vi "Launcher.vi"() -> ()   [LabVIEW 2022 SP3]
doc: "JKI State Machine Objects (SMO) 1.0.0.5\nJKI - JKI\nCopyright (c) 2016, JKI"
uses:
  002_SRC/Splashy/Splashy.lvclass
  C:/Program Files (x86)/National Instruments/LabVIEW 2022/vi.lib/JKI/JKI SMO/SMO/SMO.lvclass
  C:/Program Files (x86)/National Instruments/LabVIEW 2022/vi.lib/JKI/JKI SMO/SMO.UI/SMO.UI.lvclass
  002_SRC/GUI/GUI.lvclass
  <vilib>/JKI/JKI SMO/SMO/SMO.lvclass/SMO.ctl
  <vilib>/JKI/JKI SMO/SMO.UI/SMO.UI.lvclass/SMO.UI.ctl
  <vilib>/JKI/JKI SMO/SMO/Typedefs/SMOState --Enum.ctl
  f04c7903-df52-4a90-82d6-ebb4e2f21dec.vi
  <vilib>/JKI/JKI SMO/SMO/Private/ReftoDVR--SMO.vi
  <vilib>/JKI/JKI SMO/SMO.UI/SMO.UI.ReftoDVR.vi
  <vilib>/JKI/JKI SMO/SMO/SMO.lvclass
  <vilib>/JKI/JKI SMO/SMO.UI/SMO.UI.lvclass
  C:/Users/uib01493/Desktop/001_Final_Project/002_SRC/Splashy/Splashy.lvclass
  C:/Users/uib01493/Desktop/001_Final_Project/002_SRC/GUI/GUI.lvclass
panel:
  out "error out":errorcluster
  in  "Stop":bool
  # "SMO Splash Test Launcher"
  # "For instructions on how to use the JKI State Machine Objects, examples and video tutorials, visit:\nhttp://jki.net/state-machine-objects/\n\nJKI State Machine Objects™\nhttp://jki.net/state-machine-objects/\nCopyright (C) 2005-2015, JKI <info@jki.net>\nALL RIGHTS RESERVED"
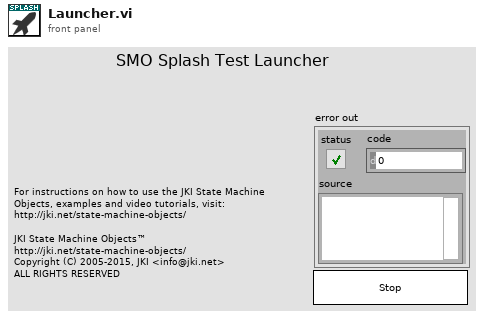
[diagram p1: front panel]
types:
  T1 = enum32{"Invalid", "Standard", "Closed", "Hidden", "Minimized", "Maximized"}
  T2 = typedef "SMO.lvclass/Public Events.ctl" = cluster{"Error":refnum<user-event>, "State":refnum<user-event>, "Reserve State":refnum<user-event>}
  T3 = typedef "SMO.UI.lvclass/PublicEvents--Cluster.ctl" = cluster{"UI Hidden":refnum<user-event>, "UI State":refnum<user-event>}
  T4 = typedef "SMO.lvclass/SMOState --Enum.ctl" = enum16{"unknown", "Created", "Started", "Stopped"}
  T5 = typedef "GUI.lvclass/PublicEvents--Cluster.ctl" = cluster{"Data Changed":refnum<user-event>}
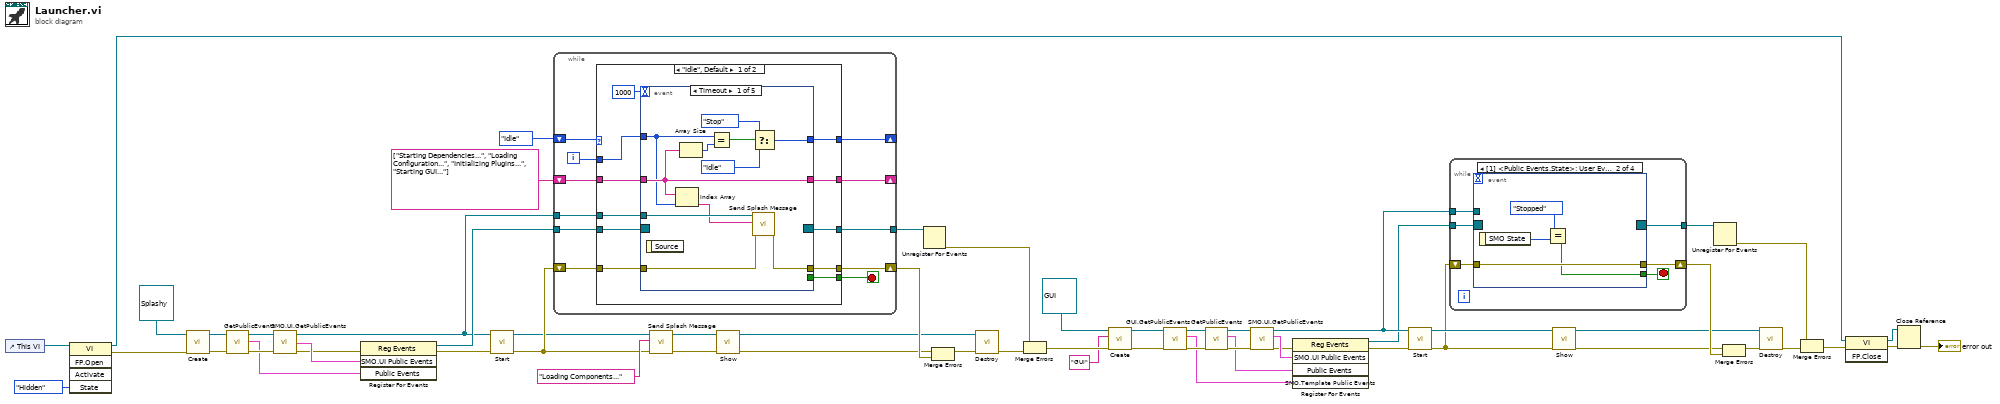
[diagram p0: block diagram]
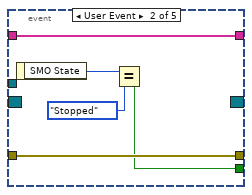
[diagram p2: hidden frame]
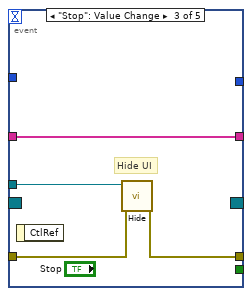
[diagram p3: hidden frame]
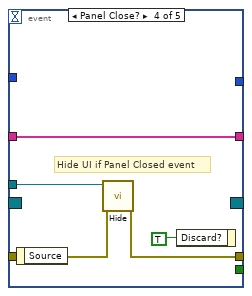
[diagram p4: hidden frame]
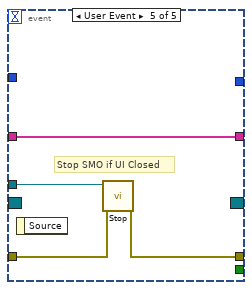
[diagram p5: hidden frame]
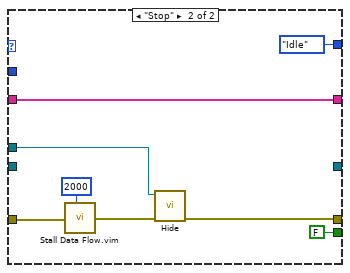
[diagram p6: hidden frame]
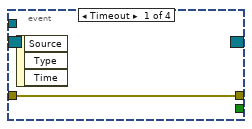
[diagram p7: hidden frame]
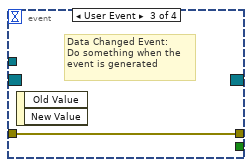
[diagram p8: hidden frame]
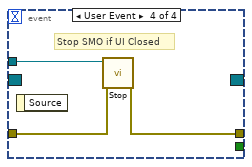
[diagram p9: hidden frame]
diagram:
  n1 = control-ref of="This VI"() -> (w8:refnum<vi>)
  n2 = invoke class="VI" method="FP.Open"(reference=w8, "State"=T1."Hidden") -> (reference out=w4:refnum<vi>, error out=w35:errorcluster)  [unwired: 3 in, 3 out]
  n3 = call <vilib>:"Create.vi"("error in (no error)"=w35, "SMO"=refnum<class "Splashy.lvclass"> refnum ("SMO.Template.lvclass")) -> ("error out"=w41:errorcluster, "SMO out"=w43:refnum<class "Splashy.lvclass">)  [unwired: 7 in, 1 out]
  n4 = call <vilib>:"GetPublicEvents.vi"("error in (no error)"=w41, "SMO"=w43) -> ("error out"=w40:errorcluster, "Public Events"=w39:T2, "SMO out"=w42:refnum<class "Splashy.lvclass">)  [unwired: 7 in]
  n5 = call <vilib>:"SMO.UI.GetPublicEvents.vi"("error in (no error)"=w40, "SMO.UI"=w42) -> ("error out"=w45:errorcluster, "SMO.UI Public Events"=w46:T3, "SMO.UI out"=w37:refnum<class "Splashy.lvclass">)  [unwired: 7 in]
  n6 = register-events(error in=w45, w46, w39) -> (reference out=w38:refnum<event-registration>, error out=w44:errorcluster)  [unwired: 1 in]
  n7 = call <vilib>:"Start.vi"("error in (no error)"=w44, "SMO"=w37) -> ("error out"=w50:errorcluster, "SMO out"=w47:refnum<class "Splashy.lvclass">)  [unwired: 8 in]
  n8 = while {
    shift-right: [w68] -> w57
    shift-left: w50 -> [w67]
    tunnel: w38 -> [w66]
    tunnel: [w65] -> w58
    tunnel: w37 -> [w64]
    shift-right: [w61] -> _
    shift-left: string[] ["Starting Dependencies...", "Loading Configuration...", "Initializing Plugins...", "Starting GUI..."] -> [w62]
    shift-right: [w60] -> _
    shift-left: enum16{"Idle", "Stop"}."Idle" -> [w59]
    i -> [w63]
    stop <- w69 stop-if-true
    n9 = case shown="\"Idle\", Default" w59 {
      tunnel: [w80 FALSE] -> w69
      tunnel: [w79 w110] -> w68
      tunnel: w67 -> [w78 w115]
      tunnel: w66 -> [w77 _]
      tunnel: [w76 _] -> w65
      tunnel: w64 -> [w75 w111]
      tunnel: w63 -> [w73 _]
      tunnel: w62 -> [w72 w116]
      tunnel: [w71 w116] -> w61
      tunnel: [w70 enum16{"Idle", "Stop"}."Idle"] -> w60
      frame "Idle", Default {
        n10 = event shown="[0] Timeout" {
          selector: w77 -> [_ _ _ _ _]
          dyn-events: [_ _ _ _ _] -> w76
          timeout: 1000 -> [_ _ _ _ _]
          tunnel: [_ w93 _ _ _] -> w80
          tunnel: w75 -> [w91 _ w100 w104 w109]
          tunnel: [w88 w96 w98 w102 w108] -> w79
          tunnel: w78 -> [w89 w96 w99 w103 w107]
          tunnel: w73 -> [w81 _ _ _ _]
          tunnel: w72 -> [w85 w92 w97 w101 w106]
          tunnel: [w85 w92 w97 w101 w106] -> w71
          tunnel: [w84 _ _ _ _] -> w70
          event Timeout {
            n11 = event-data() -> ()  [unwired: 1 in, 1 out]
            n12 = Index Array(array=w85, index=w81) -> (element=w90:string)
            n13 = Array Size(array=w85) -> (size(s)=w87:i32)
            n14 = Equal?(x=w81, y=w87) -> (x = y?=w86:bool)
            n15 = call-dynamic "Send Splash Message.vi"("error in (no error)"=w89, "Message"=w90, "Splashy"=w91) -> ("error out"=w88:errorcluster)  [unwired: 7 in, 1 out]
            n16 = Select(t=enum16{"Idle", "Stop"}."Stop", s=w86, f=enum16{"Idle", "Stop"}."Idle") -> (s? t:f=w84:enum16{"Idle", "Stop"})
          }
          event User Event {
            n17 = event-data() -> ("SMO State"=w95:T4)  [unwired: 1 in]
            n18 = Equal?(x=w95, y=SMOState_--Enum."Stopped") -> (x = y?=w93:bool)
          }
          event "Stop": Value Change {
            # "Hide UI"
            n19 = event-data() -> ()  [unwired: 1 in, 1 out]
            n20 = call <vilib>:"Hide.vi"("error in (no error)"=w99, "SMO.UI"=w100) -> ("error out"=w98:errorcluster)  [unwired: 8 in, 1 out]
          }
          event Panel Close? {
            # "Hide UI if Panel Closed event"
            n21 = event-data() -> ()  [unwired: 1 in, 1 out]
            n22 = call <vilib>:"Hide.vi"("error in (no error)"=w103, "SMO.UI"=w104) -> ("error out"=w102:errorcluster)  [unwired: 8 in, 1 out]
            n23 = event-data("Discard?"=TRUE ("OK")) -> ()  [unwired: 1 in, 1 out]
          }
          event User Event {
            # "Stop SMO if UI Closed"
            n24 = event-data() -> ()  [unwired: 1 in, 1 out]
            n25 = call <vilib>:"Stop.vi"("error in (no error)"=w107, "SMO"=w109) -> ("error out"=w108:errorcluster)  [unwired: 8 in, 1 out]
          }
        }
      }
      frame "Stop" {
        n26 = call "Stall Data Flow.vim"("value in"=w115, "milliseconds to wait"=u32 2000) -> ("value out"=w112:errorcluster)  [unwired: 1 out]
        n27 = call <vilib>:"Hide.vi"("error in (no error)"=w112, "SMO.UI"=w111) -> ("error out"=w110:errorcluster)  [unwired: 8 in, 1 out]
      }
    }
  }
  n28 = call-dynamic "Send Splash Message.vi"("error in (no error)"=w50, "Message"="Loading Components...", "Splashy"=w47) -> ("error out"=w49:errorcluster, "Splashy out"=w48:refnum<class "Splashy.lvclass">)  [unwired: 7 in]
  n29 = call <vilib>:"Show.vi"("error in (no error)"=w49, "SMO.UI"=w48) -> ("error out"=w54:errorcluster, "SMO.UI out"=w53:refnum<class "Splashy.lvclass">)  [unwired: 8 in]
  n30 = Unregister For Events(event registration refnum=w58) -> (error out=w56:errorcluster)  [unwired: 1 in]
  n31 = Merge Errors(w54, w57) -> (w52:errorcluster)
  n32 = call <vilib>:"Destroy.vi"("error in (no error)"=w52, "SMO"=w53) -> ("error out"=w32:errorcluster)  [unwired: 9 in]
  n33 = Merge Errors(w56, w32) -> (w34:errorcluster)
  n34 = call <vilib>:"Create.vi"("error in (no error)"=w34, "Subsystem Name (optional)"="GUI", "SMO"=refnum<class "GUI.lvclass"> refnum ("SMO.Template.lvclass")) -> ("error out"=w16:errorcluster, "SMO out"=w18:refnum<class "GUI.lvclass">)  [unwired: 6 in, 1 out]
  n35 = call "GUI.GetPublicEvents.vi"("error in (no error)"=w16, "GUI"=w18) -> ("error out"=w15:errorcluster, "SMO.Template Public Events"=w14:T5, "GUI out"=w17:refnum<class "GUI.lvclass">)  [unwired: 7 in]
  n36 = call <vilib>:"GetPublicEvents.vi"("error in (no error)"=w15, "SMO"=w17) -> ("error out"=w20:errorcluster, "Public Events"=w19:T2, "SMO out"=w21:refnum<class "GUI.lvclass">)  [unwired: 7 in]
  n37 = call <vilib>:"SMO.UI.GetPublicEvents.vi"("error in (no error)"=w20, "SMO.UI"=w21) -> ("error out"=w24:errorcluster, "SMO.UI Public Events"=w25:T3, "SMO.UI out"=w23:refnum<class "GUI.lvclass">)  [unwired: 7 in]
  n38 = register-events(error in=w24, w25, w19, w14) -> (reference out=w13:refnum<event-registration>, error out=w22:errorcluster)  [unwired: 1 in]
  n39 = call <vilib>:"Start.vi"("error in (no error)"=w22, "SMO"=w23) -> ("error out"=w2:errorcluster, "SMO out"=w3:refnum<class "GUI.lvclass">)  [unwired: 8 in]
  n40 = while {
    shift-right: [w122] -> w30
    shift-left: w2 -> [w121]
    tunnel: w13 -> [w120]
    tunnel: [w119] -> w31
    tunnel: w23 -> [w118]
    stop <- w123 stop-if-true
    n41 = event shown="[1] <Public Events.State>: User Event" {
      selector: w120 -> [_ _ _ _]
      dyn-events: [_ _ _ _] -> w119
      timeout: _ -> [_ _ _ _]
      tunnel: [_ w125 _ _] -> w123
      tunnel: w118 -> [_ _ _ w132]
      tunnel: [w124 w128 w129 w131] -> w122
      tunnel: w121 -> [w124 w128 w129 w130]
      event Timeout {
        n42 = event-data() -> ()  [unwired: 1 in, 3 out]
      }
      event User Event {
        n43 = event-data() -> ("SMO State"=w127:T4)  [unwired: 1 in]
        n44 = Equal?(x=SMOState_--Enum."Stopped", y=w127) -> (x = y?=w125:bool)
      }
      event User Event {
        # "Data Changed Event:\nDo something when the\nevent is generated"
        n45 = event-data() -> ()  [unwired: 1 in, 2 out]
      }
      event User Event {
        # "Stop SMO if UI Closed"
        n46 = event-data() -> ()  [unwired: 1 in, 1 out]
        n47 = call <vilib>:"Stop.vi"("error in (no error)"=w130, "SMO"=w132) -> ("error out"=w131:errorcluster)  [unwired: 8 in, 1 out]
      }
    }
  }
  n48 = call <vilib>:"Show.vi"("error in (no error)"=w2, "SMO.UI"=w3) -> ("error out"=w26:errorcluster, "SMO.UI out"=w11:refnum<class "GUI.lvclass">)  [unwired: 8 in]
  n49 = Unregister For Events(event registration refnum=w31) -> (error out=w29:errorcluster)  [unwired: 1 in]
  n50 = Merge Errors(w26, w30) -> (w12:errorcluster)
  n51 = call <vilib>:"Destroy.vi"("error in (no error)"=w12, "SMO"=w11) -> ("error out"=w28:errorcluster)  [unwired: 9 in]
  n52 = Merge Errors(w29, w28) -> (w6:errorcluster)
  n53 = invoke class="VI" method="FP.Close"(reference=w4, error in=w6) -> (reference out=w10:refnum<vi>, error out=w9:errorcluster)  [unwired: 1 in, 1 out]
  n54 = Close Reference(reference=w10, error in (no error)=w9) -> (error out=→"error out":errorcluster)
